vi "New BetterMultiListboxHandle.vi"(8 "error in (no error)":errorcluster, 10 "TreeBar Picture Ref":refnum<vi>, 11 "MCL ref":refnum<vi>) -> (0 "error out":errorcluster, 3 "BetterMultiListboxHandle out":refnum<class "BetterMultiListboxHandle.lvclass">)   [LabVIEW 2020, in "BetterDragAndDrop.lvlib" / "BetterMultiListboxHandle.lvclass"]
uses:
  BetterMultiListboxHandle.lvclass
  C:/DSCE code/Open-source/betterdraganddrop_GIT/Source/Classes/BetterHandle/BetterHandle.lvclass
  BetterMultiListboxHandle.lvclass/BetterMultiListboxHandle.ctl
  BetterHandle/BetterHandle.lvclass/BetterHandle.ctl
  BetterHandle/Write TreeBar.vi
  BetterTreeBar/BetterHorizontalBar.lvclass
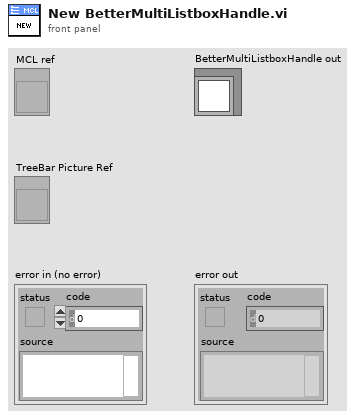
[diagram p1: front panel]
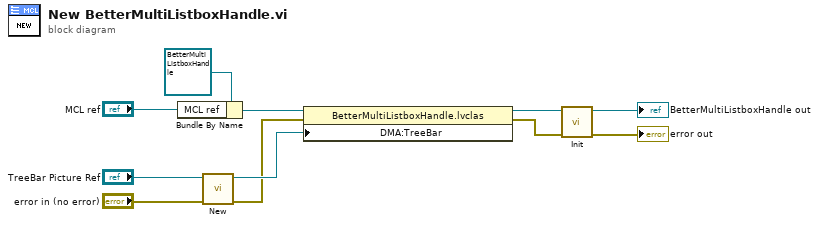
[diagram p0: block diagram]
diagram:
  n1 = Bundle By Name(cluster=refnum<class "BetterMultiListboxHandle.lvclass"> refnum ("BetterMultiListboxHandle out"), "MCL ref"="MCL ref") -> (w9:refnum<class "BetterMultiListboxHandle.lvclass">)
  n2 = call "New.vi"("error in (no error)"="error in (no error)", "Picture Ref"="TreeBar Picture Ref") -> ("error out"=w4:errorcluster, "BetterTreeBar out"=w6:refnum<class "BetterHorizontalBar.lvclass">)  [unwired: 8 in]
  n3 = property class="BetterMultiListboxHandle.lvclas"(reference=w9, error in=w4, "DMA:TreeBar"=w6) -> (reference out=w5:refnum<class "BetterMultiListboxHandle.lvclass">, error out=w3:errorcluster)
  n4 = call-dynamic "Init.vi"("error in (no error)"=w3, "BetterMultiListboxHandle in"=w5) -> ("error out"=→"error out":errorcluster, "BetterMultiListboxHandle out"=→"BetterMultiListboxHandle out":refnum<class "BetterMultiListboxHandle.lvclass">)  [unwired: 8 in]
